vi "Forces Set.vi"(8 "error in (no error)":errorcluster, 10 "Forces":T1) -> (0 "error out":errorcluster)   [LabVIEW 2019, in "Haptic Prog Interface.lvlib"]
doc: "Returns the forces of the haptic pen in N.\n\n<b>Position:</b> Returns a cluster of the x, y, and z forces on the pen (in units of N)."
uses:
  Haptic Prog Interface.lvlib
  dll_path.vi
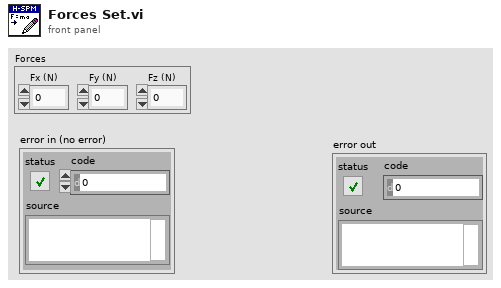
[diagram p1: front panel]
types:
  T1 = cluster{"Fx (N)":dbl, "Fy (N)":dbl, "Fz (N)":dbl}
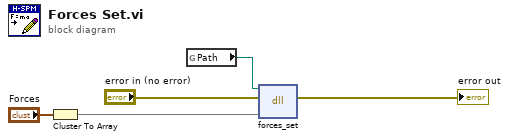
[diagram p0: block diagram]
diagram:
  n1 = Cluster To Array(cluster="Forces") -> (array=w1:dbl[])
  n2 = global read "dll_path.vi" "Path"() -> (w5:path)
  n3 = dll-call lib="C:/Users/freem/Documents/GitHub/HapticSPM/Haptic-Programming-Interface/x64/Debug/Haptic Programming Interface.dll" fn="forces_set"(path in=w5, error in="error in (no error)", "input"=w1) -> (error out=→"error out":errorcluster)  [unwired: 3 in, 1 out]
